vi "Controlword_ReadMode.vi"(10 "Read mode":T1, 11 "ControlWord In":u16 format="%08b") -> (3 "ControlWord Out":u16 format="%08b")   [LabVIEW 2017, in "WordManipulationLibrary.lvlib"]
uses:
  WordManipulationLibrary.lvlib
  Controlword_ReadMode.ctl
  Bit Manipulation.lvlib
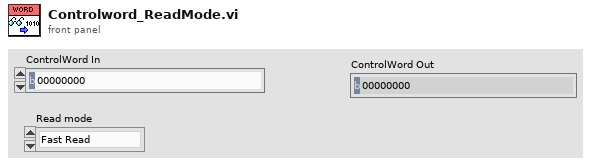
[diagram p1: front panel]
types:
  T1 = typedef "WordManipulationLibrary.lvlib/Controlword_ReadMode.ctl" = enum16{"Fast Read", "Full Read", "Full Read With Fault Check"}
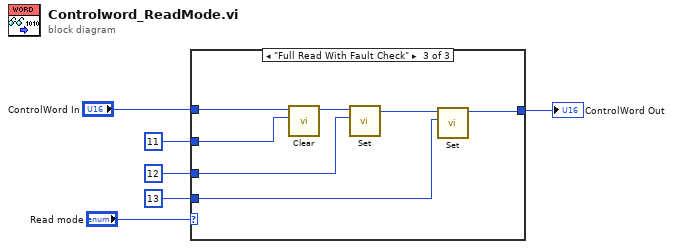
[diagram p0: block diagram]
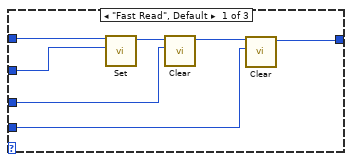
[diagram p2: hidden frame]
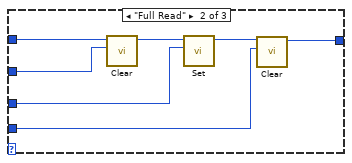
[diagram p3: hidden frame]
diagram:
  n1 = case shown="\"Full Read With Fault Check\"" "Read mode" {
    tunnel: "ControlWord In" -> [w13 w20 w27]
    tunnel: [w8 w15 w22] -> w4
    tunnel: u8 11 ("Bit to set") -> [w11 w18 w25]
    tunnel: u8 12 ("Bit to set") -> [w10 w17 w24]
    tunnel: u8 13 ("Bit to set") -> [w7 w14 w21]
    frame "Fast Read", Default {
      n2 = call "Set.vi"("Bit to set"=w11, "Data_In"=w13) -> ("Data_Out"=w12:u16)  [unwired: 9 in]
      n3 = call "Clear.vi"("Bit to clear"=w10, "Data_In"=w12) -> ("Data_Out"=w9:u16)  [unwired: 9 in]
      n4 = call "Clear.vi"("Bit to clear"=w7, "Data_In"=w9) -> ("Data_Out"=w8:u16)  [unwired: 9 in]
    }
    frame "Full Read" {
      n5 = call "Clear.vi"("Bit to clear"=w18, "Data_In"=w20) -> ("Data_Out"=w19:u16)  [unwired: 9 in]
      n6 = call "Set.vi"("Bit to set"=w17, "Data_In"=w19) -> ("Data_Out"=w16:u16)  [unwired: 9 in]
      n7 = call "Clear.vi"("Bit to clear"=w14, "Data_In"=w16) -> ("Data_Out"=w15:u16)  [unwired: 9 in]
    }
    frame "Full Read With Fault Check" {
      n8 = call "Clear.vi"("Bit to clear"=w25, "Data_In"=w27) -> ("Data_Out"=w26:u16)  [unwired: 9 in]
      n9 = call "Set.vi"("Bit to set"=w24, "Data_In"=w26) -> ("Data_Out"=w23:u16)  [unwired: 9 in]
      n10 = call "Set.vi"("Bit to set"=w21, "Data_In"=w23) -> ("Data_Out"=w22:u16)  [unwired: 9 in]
    }
  }
  "ControlWord Out" <- w4
